vi "test2-testModuleTurnsInvalidAPI.vi"(8 "error in (no error)":errorcluster, 11 "TestCase in":refnum<class "testcase-CSMNonCSMCallerSupportAPI.lvclass">) -> (0 "error out":errorcluster, 3 "TestCase out":refnum<class "testcase-CSMNonCSMCallerSupportAPI.lvclass">)   [LabVIEW 2017, in "testcase-CSMNonCSMCallerSupportAPI.lvclass"]
uses:
  testcase-CSMNonCSMCallerSupportAPI.lvclass
  InternalCluster.ctl
  GlobalVariable_CSMModeData.vi
  src/user.lib/_NEVSTOP/Communicable State Machine(CSM)/AdvanceAPI/CSM - List Modules.vi
  <vilib>/addons/_JKI Toolkits/VI Tester/TestCase.llb/TestCase.lvclass
  src/user.lib/_NEVSTOP/Communicable State Machine(CSM)/Communicable State Machine.lvlib
  CSM/CSM-Testcase.lvlib
  C:/Program Files (x86)/National Instruments/LabVIEW 2017/vi.lib/addons/_JKI Toolkits/VI Tester/TestCase.llb/TestCase.lvclass
panel:
  in  "Stop":bool
  out "LoopCount":i32
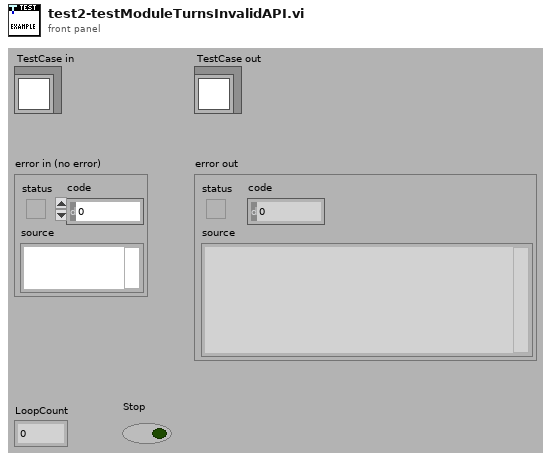
[diagram p1: front panel]
types:
  T1 = typedef "testcase-CSMNonCSMCallerSupportAPI.lvclass/InternalCluster.ctl" = cluster{"Mode":enum16{"Invalid", "Others", "WorkerAgent or Chain"}, "#Nodes":u32}
  T2 = enum16{"Invalid", "Others", "WorkerAgent or Chain"}
  T3 = typedef "Communicable State Machine.lvlib/_CSM_MODE.ctl" = enum16{"Not Exist", "Stand Alone", "CSM", "Worker", "Worker Agent", "Chain Node", "Chain"}
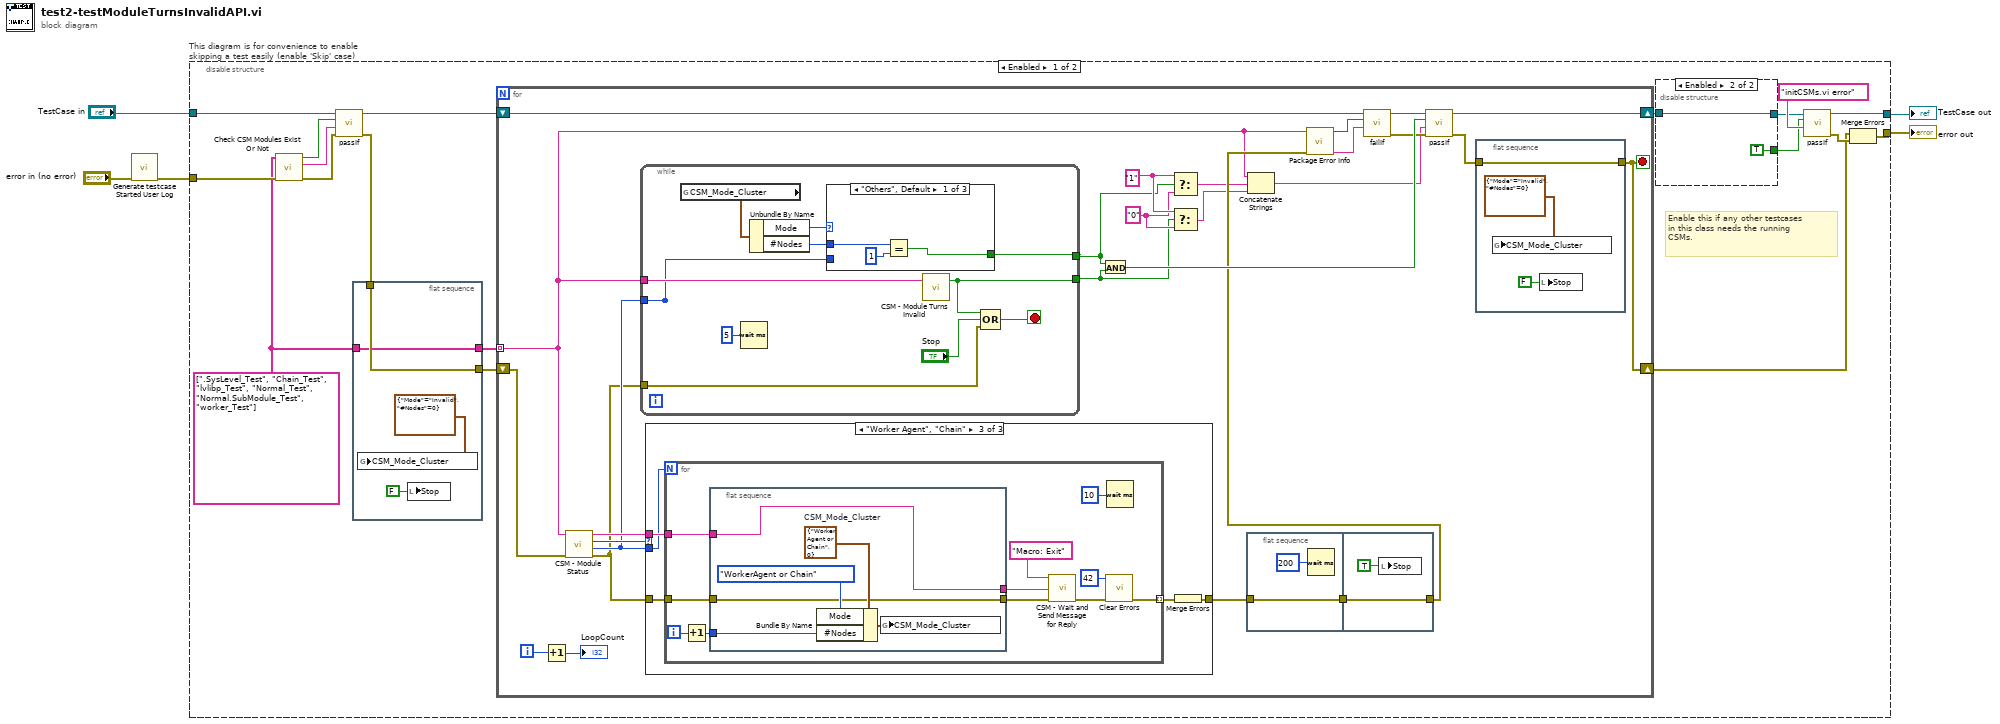
[diagram p0: block diagram]
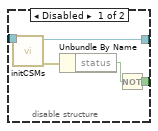
[diagram p2: hidden frame]
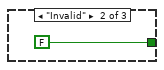
[diagram p3: hidden frame]
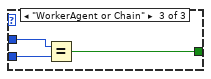
[diagram p4: hidden frame]
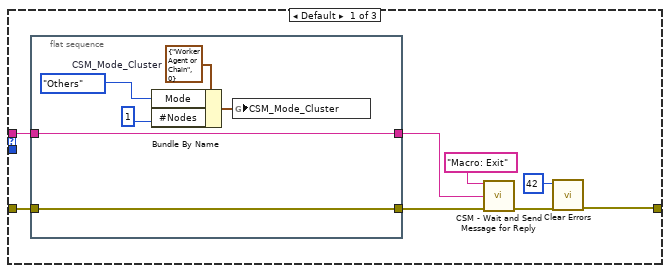
[diagram p5: hidden frame]
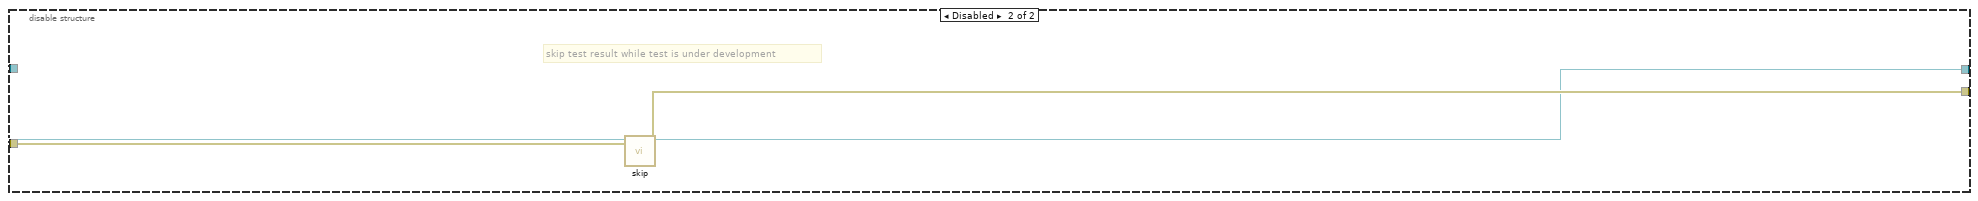
[diagram p7: hidden frame]
diagram:
  n1 = call "Generate testcase Started User Log.vi"("Error In"="error in (no error)") -> ("error out"=w1:errorcluster)  [unwired: 10 in]
  n2 = disable-structure "This diagram is for convenience to enable skipping a test easily (enable 'Skip' case)" shown="Enabled" {
    disable-tunnel: "TestCase in" -> [w19 w127]
    disable-tunnel: [w9 w125] -> w2
    disable-tunnel: [w7 w126] -> w4
    disable-tunnel: w1 -> [w17 w124]
    frame Enabled {
      w6 = string[] [".SysLevel_Test", "Chain_Test", "lvlibp_Test", "Normal_Test", "Normal.SubModule_Test", "worker_Test"] ("Module Names in All Scope")
      # "Enable this if any other testcases \nin this class needs the running\nCSMs."
      n3 = call "Check CSM Modules Exist Or Not.vi"("error in"=w17, "CSM names in"=w6) -> ("error out"=w21:errorcluster, "Debug string"=w22:string, "All Modules Exist?"=w23:bool)  [unwired: 7 in]
      n4 = call-dynamic "passIf.vi"("error in (no error)"=w21, "message (\"\")"=w22, "pass"=w23, "TestCase in"=w19) -> ("error out"=w20:errorcluster, "TestCase out"=w18:refnum<class "testcase-CSMNonCSMCallerSupportAPI.lvclass">)  [unwired: 6 in]
      n5 = flat-sequence {
        tunnel: [w32] -> w16
        tunnel: [w31] -> w15
        tunnel: w20 -> [w32]
        tunnel: w6 -> [w31]
        frame #0 {
          n6 = global write "GlobalVariable_CSMModeData.vi" "CSM_Mode_Cluster"(T1 {"Mode"=enum."Invalid", "#Nodes"=0} ("CSM_Mode_Cluster")) -> ()
          n7 = local write "Stop"(FALSE ("Stop")) -> ()
        }
      }
      n8 = for {
        shift-right: [w49] -> w8
        shift-left: w16 -> [w59]
        shift-right: [w56] -> w10
        shift-left: w18 -> [w46]
        tunnel: w15 -> [w36] mode=indexing
        i -> [w61]
        stop <- w49 stop-if-true
        w41 = "0"
        w42 = "1"
        n9 = Increment(x=w61) -> (x+1=→"LoopCount":i32)
        n10 = call "CSM - Module Status.vi"("Error In"=w59, "CSM Name"=w36) -> ("error out"=w50:errorcluster, "#Nodes"=w52:i32, "Mode"=w58:T3, "CSM Name (Dup)"=w57:string)  [unwired: 5 in, 1 out]
        n11 = while {
          tunnel: w36 -> [w76]
          tunnel: [w70] -> _
          tunnel: w52 -> [w70]
          tunnel: [w69] -> w37
          tunnel: [w68] -> w38
          tunnel: w50 -> [w67]
          stop <- w74 stop-if-true
          n12 = global read "GlobalVariable_CSMModeData.vi" "CSM_Mode_Cluster"() -> (w73:T1)
          n13 = Wait (ms)(milliseconds to wait=u32 5) -> ()  [unwired: 1 out]
          n14 = Unbundle By Name(w73) -> ("Mode"=w72:T2, "#Nodes"=w71:u32)
          n15 = case shown="\"Others\", Default" w72 {
            tunnel: [w79 FALSE w82] -> w68
            tunnel: w71 -> [w78 _ w83]
            tunnel: w70 -> [_ _ w81]
            frame "Others", Default {
              n16 = Equal?(x=w78, y=1) -> (x = y?=w79:bool)
            }
            frame "Invalid" {
            }
            frame "WorkerAgent or Chain" {
              n17 = Equal?(x=w83, y=w81) -> (x = y?=w82:bool)
            }
          }
          n18 = call "CSM - Module Turns Invalid.vi"("CSM Name"=w76) -> ("Turn Invalid (Exit)?"=w69:bool)  [unwired: 2 in]
          n19 = Compound Arithmetic op=OR(w69, "Stop", w67) -> (w74:bool)
        }
        n20 = case shown="\"Worker Agent\", \"Chain\"" w58 {
          tunnel: w50 -> [w88 w101 w106]
          tunnel: w52 -> [_ _ w104]
          tunnel: w57 -> [w90 _ w105]
          tunnel: [w92 w101 w103] -> w54
          frame Default {
            n21 = flat-sequence {
              tunnel: w90 -> [w96]
              tunnel: [w96] -> w89
              tunnel: w88 -> [w95]
              tunnel: [w95] -> w87
              frame #0 {
                w100 = T1 {"Mode"=enum."WorkerAgent or Chain", "#Nodes"=0}  # CSM_Mode_Cluster
                n22 = Bundle By Name(cluster=w100, "Mode"=T2."Others", "#Nodes"=u32 1) -> (w99:T1)
                n23 = global write "GlobalVariable_CSMModeData.vi" "CSM_Mode_Cluster"(w99) -> ()
              }
            }
            n24 = call "CSM - Wait and Send Message for Reply.vi"("State"="Macro: Exit", "Target Module"=w89, "Error In (No Error)"=w87) -> ("error out"=w93:errorcluster)  [unwired: 9 in, 3 out]
            n25 = call <vilib>:"Clear Errors.vi"("error in (no error)"=w93, "specific error code to clear (0: all)"=42) -> ("error out"=w92:errorcluster)  [unwired: 4 in, 1 out]
          }
          frame "Not Exist" {
          }
          frame "Worker Agent", "Chain" {
            n26 = for {
              N: w104 -> [_]
              tunnel: w105 -> [w108]
              tunnel: w106 -> [w110]
              tunnel: [w113] -> w102 mode=indexing
              i -> [w116]
              n27 = Increment(x=w116) -> (x+1=w115:i32)
              n28 = flat-sequence {
                tunnel: w115 -> [w121]
                tunnel: w110 -> [w119]
                tunnel: [w119] -> w109
                tunnel: w108 -> [w118]
                tunnel: [w118] -> w107
                frame #0 {
                  w123 = T1 {"Mode"=enum."WorkerAgent or Chain", "#Nodes"=0}  # CSM_Mode_Cluster
                  n29 = Bundle By Name(cluster=w123, "Mode"=T2."WorkerAgent or Chain", "#Nodes"=w121) -> (w122:T1)
                  n30 = global write "GlobalVariable_CSMModeData.vi" "CSM_Mode_Cluster"(w122) -> ()
                }
              }
              n31 = call "CSM - Wait and Send Message for Reply.vi"("State"="Macro: Exit", "Target Module"=w107, "Error In (No Error)"=w109) -> ("error out"=w114:errorcluster)  [unwired: 9 in, 3 out]
              n32 = call <vilib>:"Clear Errors.vi"("error in (no error)"=w114, "specific error code to clear (0: all)"=42) -> ("error out"=w113:errorcluster)  [unwired: 4 in, 1 out]
              n33 = Wait (ms)(milliseconds to wait=u32 10) -> ()  [unwired: 1 out]
            }
            n34 = Merge Errors(w102) -> (w103:errorcluster)
          }
        }
        n35 = And(x=w38, y=w37) -> (x .and. y?=w51:bool)
        n36 = Select(t=w42, s=w38, f=w41) -> (s? t:f=w40:string)
        n37 = Select(t=w42, s=w37, f=w41) -> (s? t:f=w39:string)
        n38 = flat-sequence {
          tunnel: w54 -> [w63]
          tunnel: [w63] -> w53
          tunnel: [w65] -> w43
          tunnel: w53 -> [w65]
          frame #0 {
            n39 = Wait (ms)(milliseconds to wait=u32 200) -> ()  [unwired: 1 out]
          }
          frame #1 {
            n40 = local write "Stop"(TRUE ("Stop")) -> ()
          }
        }
        n41 = Concatenate Strings(w36, w40, w39) -> (w35:string)
        n42 = call "Package Error Info.vi"("error in"=w43, "String in"=w36) -> ("packed error info out"=w47:string, "error status"=w48:bool)  [unwired: 8 in]
        n43 = call-dynamic "failIf.vi"("message (\"\")"=w47, "fail"=w48, "TestCase in"=w46) -> ("error out"=w44:errorcluster, "TestCase out"=w45:refnum<class "testcase-CSMNonCSMCallerSupportAPI.lvclass">)  [unwired: 7 in]
        n44 = call-dynamic "passIf.vi"("error in (no error)"=w44, "message (\"\")"=w35, "pass"=w51, "TestCase in"=w45) -> ("error out"=w55:errorcluster, "TestCase out"=w56:refnum<class "testcase-CSMNonCSMCallerSupportAPI.lvclass">)  [unwired: 6 in]
        n45 = flat-sequence {
          tunnel: w55 -> [w85]
          tunnel: [w85] -> w49
          frame #0 {
            n46 = global write "GlobalVariable_CSMModeData.vi" "CSM_Mode_Cluster"(T1 {"Mode"=enum."Invalid", "#Nodes"=0} ("CSM_Mode_Cluster")) -> ()
            n47 = local write "Stop"(FALSE ("Stop")) -> ()
          }
        }
      }
      n48 = disable-structure shown="Enabled" {
        disable-tunnel: [w28 TRUE ("pass")] -> w13
        disable-tunnel: [w25 w30] -> w12
        disable-tunnel: w10 -> [w24 w30]
        frame Disabled {
          n49 = call "initCSMs.vi"("TestCase in"=w24) -> ("error out"=w26:errorcluster, "TestCase out"=w25:refnum<class "testcase-CSMNonCSMCallerSupportAPI.lvclass">)  [unwired: 9 in]
          n50 = Unbundle By Name(w26) -> ("status"=w27:bool)
          n51 = Not(x=w27) -> (.not. x?=w28:bool)
        }
        frame Enabled {
        }
      }
      n52 = call-dynamic "passIf.vi"("message (\"\")"="initCSMs.vi error" ("message (\"\")"), "pass"=w13, "TestCase in"=w12) -> ("error out"=w11:errorcluster, "TestCase out"=w9:refnum<class "testcase-CSMNonCSMCallerSupportAPI.lvclass">)  [unwired: 7 in]
      n53 = Merge Errors(w8, w11) -> (w7:errorcluster)
    }
    frame Disabled {
      # "skip test result while test is under development"
      n54 = call <vilib>:"skip.vi"("error in (no error)"=w124, "TestCase in"=w127) -> ("error out"=w126:errorcluster, "TestCase out"=w125:refnum<class "testcase-CSMNonCSMCallerSupportAPI.lvclass">)  [unwired: 8 in]
    }
  }
  "error out" <- w4
  "TestCase out" <- w2
